vi "prime and drain.vi"() -> ()   [LabVIEW 2014]
panel:
  out "Stop Drain":bool
  in  "Stop Button":bool
  out "Boolean":bool=TRUE
  out "Prime":bool
  in  "Drain":bool
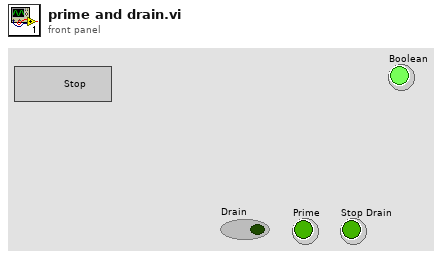
[diagram p1: front panel]
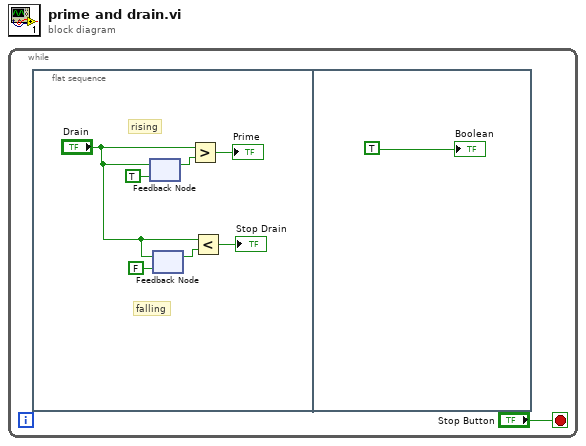
[diagram p0: block diagram]
diagram:
  n1 = while {
    stop <- "Stop Button" stop-if-true
    n2 = flat-sequence {
      frame #0 {
        # "falling"
        # "rising"
        n3 = feedback #1(TRUE ("DrainPumpRelay")) -> (w7:bool)
        n4 = feedback-in #1("Drain") -> ()
        n5 = feedback #2(FALSE ("DrainPumpRelay")) -> (w5:bool)
        n6 = feedback-in #2("Drain") -> ()
        n7 = Greater?(x="Drain", y=w7) -> (0:→"Prime":bool)
        n8 = Less?(x="Drain", y=w5) -> (x < y?=→"Stop Drain":bool)
      }
      frame #1 {
        "Boolean" <- TRUE
      }
    }
  }
